vi "Is Valid.vi"(8 "error in":errorcluster, 11 "CFG Base in":refnum<class "CFG Base.lvclass">) -> (0 "error out":errorcluster, 2 "Valid":bool, 3 "CFG Base out":refnum<class "CFG Base.lvclass">)   [LabVIEW 2023, in "HAL.lvlib" / "CFG Base.lvclass"]
uses:
  CFG Base.lvclass
  CFG Base.lvclass/CFG Base.ctl
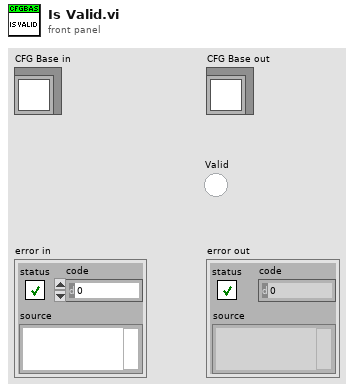
[diagram p1: front panel]
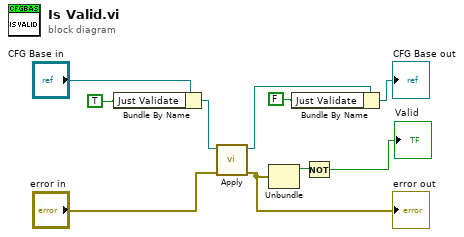
[diagram p0: block diagram]
diagram:
  n1 = Bundle By Name(cluster="CFG Base in", "Just Validate"=TRUE) -> (w8:refnum<class "CFG Base.lvclass">)
  n2 = call-dynamic "Apply.vi"("error in"="error in", "CFG Base in"=w8) -> ("error out"=w6:errorcluster, "CFG Base out"=w3:refnum<class "CFG Base.lvclass">)  [unwired: 8 in]
  "error out" <- w6
  n3 = Unbundle(w6) -> ("status"=w5:bool)  [unwired: 2 out]
  n4 = Bundle By Name(cluster=w3, "Just Validate"=FALSE) -> (→"CFG Base out":refnum<class "CFG Base.lvclass">)
  n5 = Not(x=w5) -> (.not. x?=→"Valid":bool)
